vi "9x9 find.vi"(1 "9x9  input":i32[][](array[numeric]), 2 "1~9 input":i32[](array[numeric])) -> (0 "1~9  output":i32[](array[numeric]))   [LabVIEW 2014]
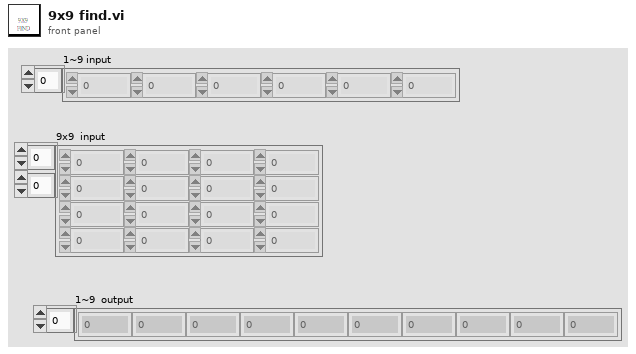
[diagram p1: front panel]
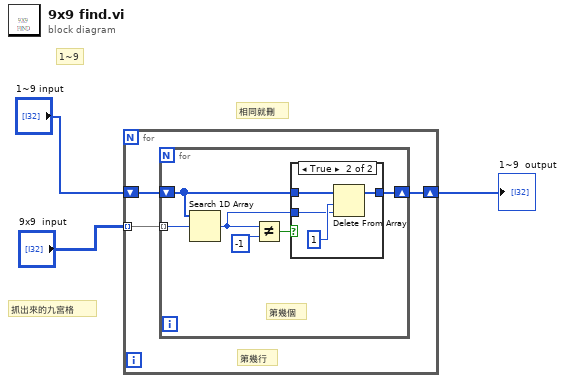
[diagram p0: block diagram]
diagram:
  # "相同就刪"
  # "抓出來的九宮格"
  # "1~9"
  n1 = for {
    tunnel: "9x9  input" -> [w6] mode=indexing
    shift-right: [w4] -> w1
    shift-left: "1~9 input" -> [w5]
    # "第幾行"
    n2 = for {
      tunnel: w6 -> [w12] mode=indexing
      shift-right: [w8] -> w4
      shift-left: w5 -> [w7]
      # "第幾個"
      n3 = Search 1D Array(1D array=w7, element=w12) -> (index of element=w9:i32)  [unwired: 1 in]
      n4 = Not Equal?(x=w9, y=-1) -> (x != y?=w10:bool)
      n5 = case shown="True" w10 {
        tunnel: w7 -> [w13 w17]
        tunnel: w9 -> [_ w15]
        tunnel: [w13 w14] -> w8
        frame False {
        }
        frame True {
          n6 = Delete From Array(array=w17, length=1, index=w15) -> (array with subset deleted=w14:i32[])  [unwired: 1 out]
        }
      }
    }
  }
  "1~9  output" <- w1
